vi "Convert Phasor Array to g & s Arrays.vi"(2 "Phasor Array":T1[](array[typedef])) -> (7 "g":dbl[](array[numeric]), 9 "s":dbl[](array[numeric]))   [LabVIEW 2019]
uses:
  Phasor (g, s).ctl
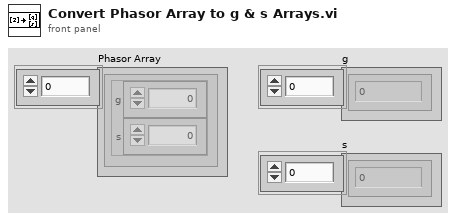
[diagram p1: front panel]
types:
  T1 = typedef "Phasor (g, s).ctl" = cluster{"g":dbl, "s":dbl}
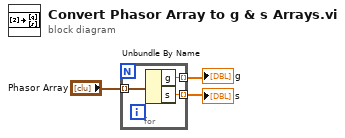
[diagram p0: block diagram]
diagram:
  n1 = for {
    tunnel: "Phasor Array" -> [w6] mode=indexing
    tunnel: [w5] -> w2 mode=indexing
    tunnel: [w4] -> w1 mode=indexing
    n2 = Unbundle By Name(w6) -> ("g"=w4:dbl, "s"=w5:dbl)
  }
  "s" <- w2
  "g" <- w1
